vi "Library_Swimbladder_init.vi"(8 "error in (no error)":errorcluster) -> (0 "error out":errorcluster)   [LabVIEW 2013]
uses:
  My Computer/Controls/Swimbladder Tuning Parameters.ctl
  My Computer/Controls/Advanced Swimbladder Indicators.ctl
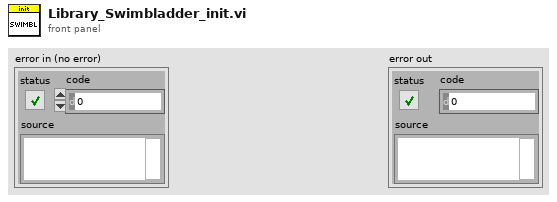
[diagram p1: front panel]
types:
  T1 = typedef "Advanced Swimbladder Indicators.ctl" = cluster{"P_ref [Pa]":dbl, "X_Actual [m]":dbl, "Motor Current[A]":dbl}
  T2 = typedef "Swimbladder Tuning Parameters.ctl" = cluster{"Excessive_Depth_Deviation_Trigger":dbl, "Neutral Buoancy_x":dbl, "Ti_Depth_Control":dbl, "kp_Depth_Control":dbl, "Integrator enabled range Depth":dbl, "Integrator_enable_Range_Motor":dbl, "kp_Motor":dbl, "Ti_Motor":dbl}
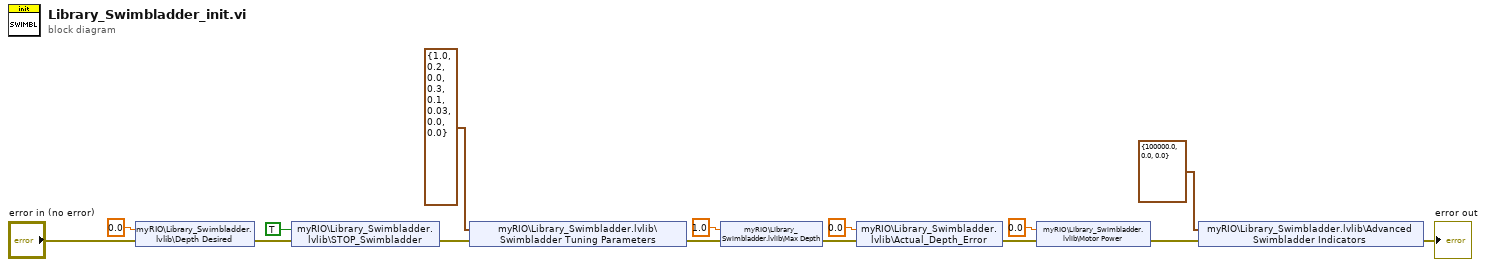
[diagram p0: block diagram]
diagram:
  n1 = shared-variable "myRIO\\Library_Swimbladder.lvlib\\Depth Desired"(0.0 ("Depth Desired"), error in="error in (no error)") -> (error out=w8:errorcluster)
  n2 = shared-variable "myRIO\\Library_Swimbladder.lvlib\\STOP_Swimbladder"(TRUE ("STOP_Swimbladder"), error in=w8) -> (error out=w7:errorcluster)
  n3 = shared-variable "myRIO\\Library_Swimbladder.lvlib\\Swimbladder Tuning Parameters"(T2 {"Excessive_Depth_Deviation_Trigger"=1.0, "Neutral Buoancy_x"=0.2, "Ti_Depth_Control"=0.0, "kp_Depth_Control"=0.3, "Integrator enabled range Depth"=0.1, "Integrator_enable_Range_Motor"=0.03, "kp_Motor"=0.0, "Ti_Motor"=0.0} ("Swimbladder Tuning Parameters"), error in=w7) -> (error out=w6:errorcluster)
  n4 = shared-variable "myRIO\\Library_Swimbladder.lvlib\\Max Depth"(1.0 ("Max Depth"), error in=w6) -> (error out=w5:errorcluster)
  n5 = shared-variable "myRIO\\Library_Swimbladder.lvlib\\Actual_Depth_Error"(0.0 ("Actual_Depth_Error"), error in=w5) -> (error out=w4:errorcluster)
  n6 = shared-variable "myRIO\\Library_Swimbladder.lvlib\\Motor Power"(0.0 ("Motor Power"), error in=w4) -> (error out=w3:errorcluster)
  n7 = shared-variable "myRIO\\Library_Swimbladder.lvlib\\Advanced Swimbladder Indicators"(T1 {"P_ref [Pa]"=100000.0, "X_Actual [m]"=0.0, "Motor Current[A]"=0.0} ("Advanced Swimbladder Indicators"), error in=w3) -> (error out=→"error out":errorcluster)
